vi "Clear Data.vi"(8 "error in (no error)":errorcluster, 11 "Model in":refnum<class "Model.lvclass">) -> (0 "error out":errorcluster, 3 "Model out":refnum<class "Model.lvclass">)   [LabVIEW 2016, in "Model.lvclass"]
uses:
  Model.lvclass
  Typedefs/ToveyEngData.ctl
  Typedefs/ActuatorData.ctl
  Typedefs/ActuatorSetPoints.ctl
  Model.lvclass/Model.ctl
  Typedefs/FAMT Typedefs.lvlib
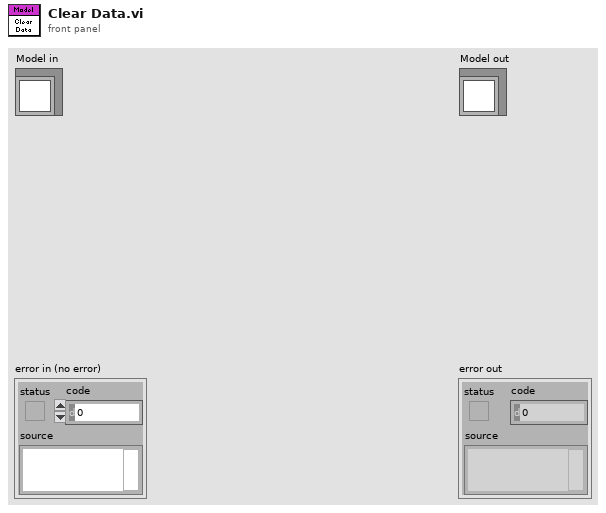
[diagram p1: front panel]
types:
  T1 = typedef "FAMT Typedefs.lvlib/ActuatorSetPoints.ctl" = cluster{"Axial Force":dbl, "Lateral Force":dbl, "FC1 Force":dbl, "FC2 Force":dbl}
  T2 = typedef "FAMT Typedefs.lvlib/ActuatorData.ctl" = cluster{"Timestamp":dbl, "Axial Force":dbl, "Lateral Force":dbl, "FC1 Force":dbl, "FC2 Force":dbl, "Lateral Push Pressure":dbl, "Lateral Pull Pressure":dbl, "Axial Push Pressure":dbl, "Axial Pull Pressure":dbl}
  T3 = typedef "FAMT Typedefs.lvlib/ToveyEngData.ctl" = cluster{"Timestamp":dbl, "Fx":dbl, "Fy":dbl, "Fz":dbl, "Mx":dbl, "My":dbl, "Mz":dbl}
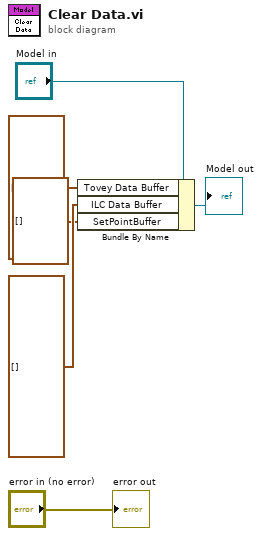
[diagram p0: block diagram]
diagram:
  n1 = Bundle By Name(cluster="Model in", "Tovey Data Buffer"=T3[] [] ("ToveyData"), "ILC Data Buffer"=T2[] [] ("ILCData"), "SetPointBuffer"=T1[] []) -> (→"Model out":refnum<class "Model.lvclass">)
  "error out" <- "error in (no error)"
